vi "arduino_FSM.vi"() -> ()   [LabVIEW 2019]
uses:
  <vilib>/Instr/_visa.llb/VISA Configure Serial Port (Instr).vi
panel:
  out "Boolean":bool
  out "Waveform Chart":dbl(graph)
  out "Response":string
  in  "Output Current [A]":dbl(knob) max=1.0 scale=0.0..1.0 scale format="%#_4g"
  in  "Output Voltage [V]":dbl(knob) max=12.0 scale=12.0..15.0
  in  "DC Power Supply Settings":T1 {"Range" items=["P25V", "P6V", "N25V"]}
  in  "STOP":bool
  in  "Command":string="*IDN?"
  in  "Read Count":u32=1000
  in  "Write":bool
  in  "Read":bool
  in  "Serial Communication Settings":T2={"Port"="", "baud rate"=9600} {"baud rate" items=["75"=75, "110"=110, "134"=134, "150"=150, "300"=300, "600"=600, "1200"=1200, "1800"=1800, "2400"=2400, "4800"=4800, "7200"=7200, "9600"=9600, "14400"=14400, "19200"=19200, "28800"=28800, "38400"=38400, "56000"=56000, "57600"=57600, "115200"=115200, "128000"=128000, "230400"=230400]}
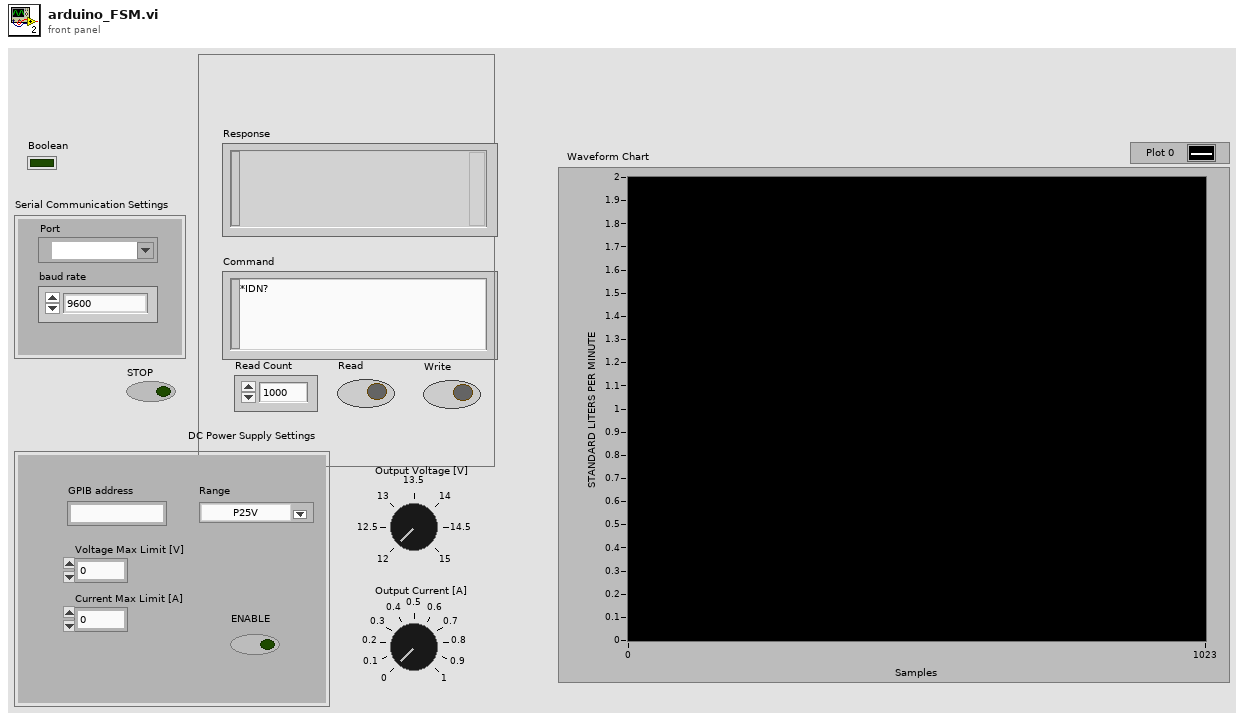
[diagram p1: front panel]
types:
  T1 = cluster{"GPIB address":string, "Range":u16, "Voltage Max Limit [V]":dbl, "Current Max Limit [A]":dbl, "ENABLE":bool}
  T2 = cluster{"Port":refnum<visa-resource-name>, "baud rate":u32}
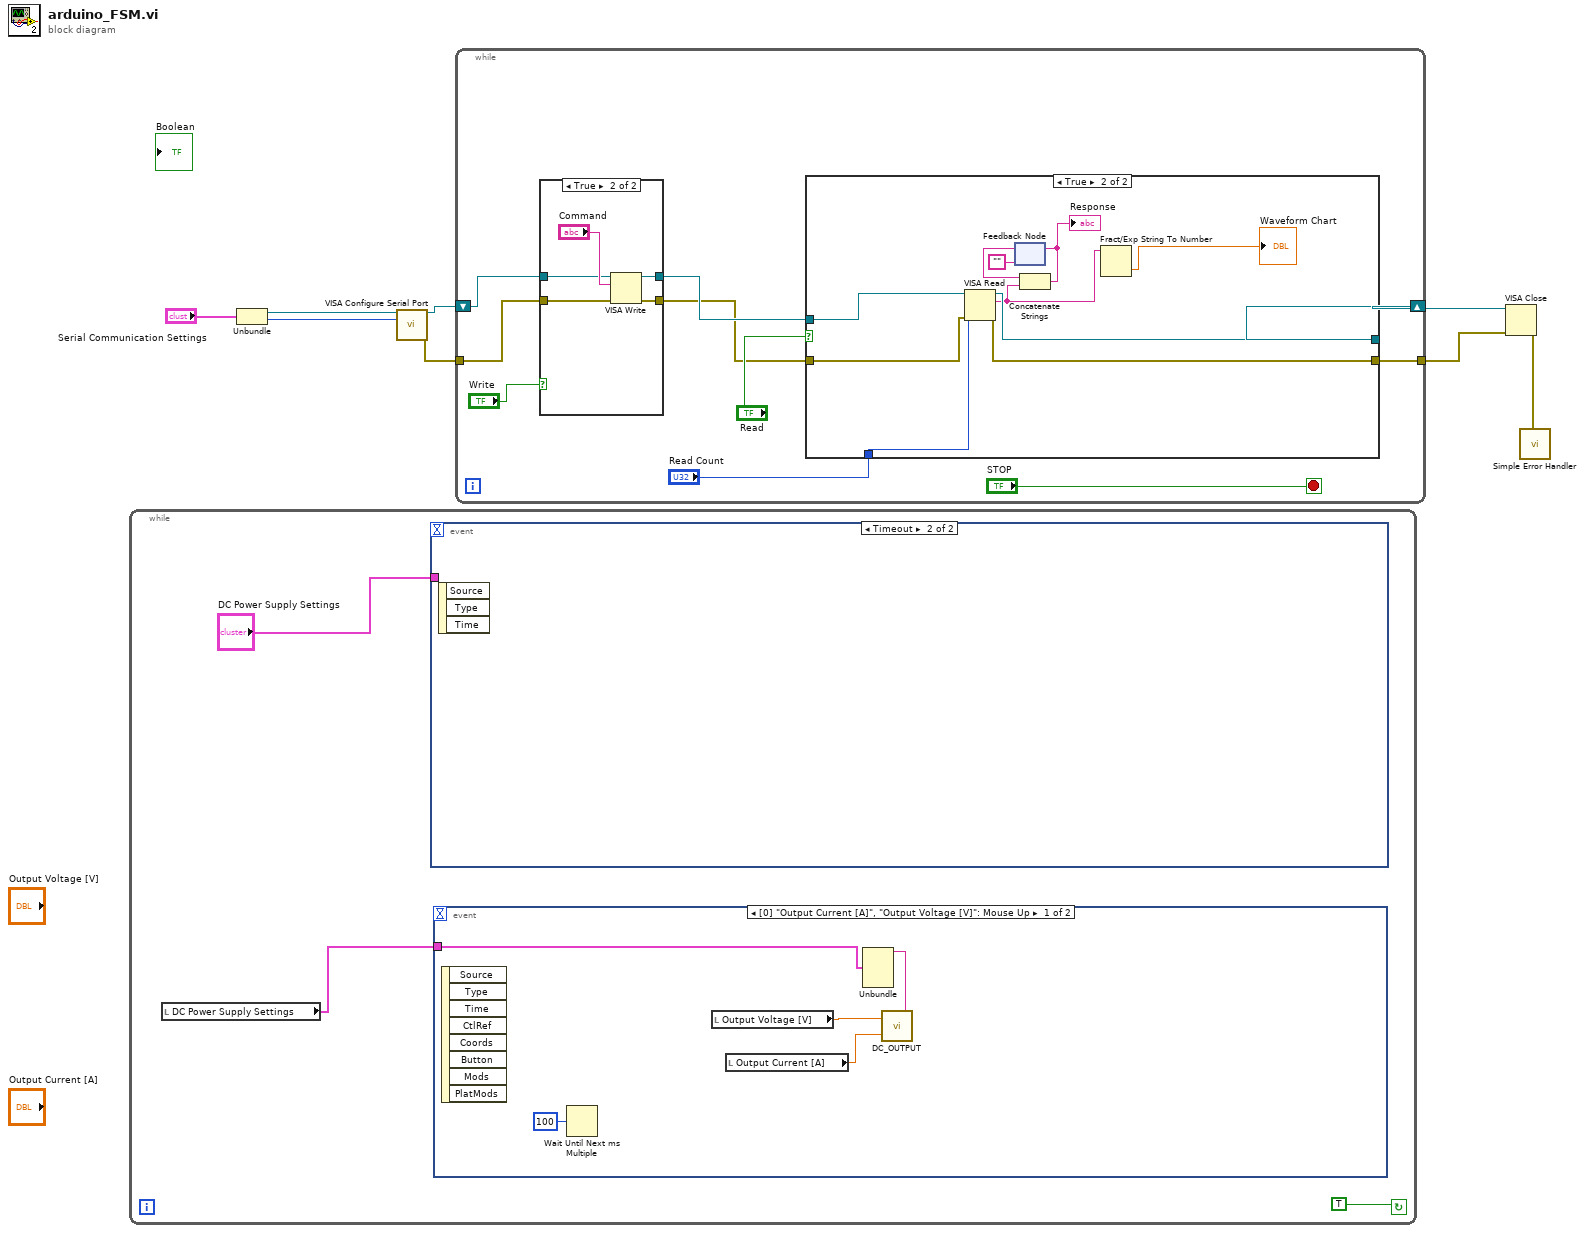
[diagram p0: block diagram]
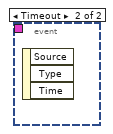
[diagram p2: hidden frame]
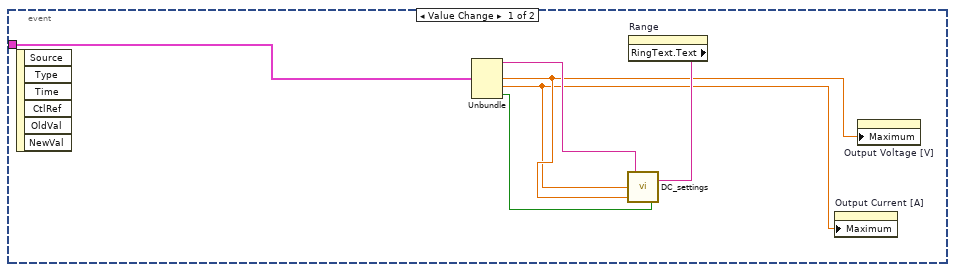
[diagram p3: hidden frame]
diagram:
  n1 = while {
    stop <- TRUE continue-if-true
    n2 = local read "DC Power Supply Settings"() -> (w10:T1)
    n3 = event shown="[1] Timeout" {
      selector: _ -> [_ _]
      dyn-events: _ -> [_ _]
      timeout: _ -> [_ _]
      tunnel: "DC Power Supply Settings" -> [w17 _]
      event "DC Power Supply Settings.ENABLE": Value Change {
        n4 = event-data() -> ()  [unwired: 1 in, 6 out]
        n5 = Unbundle(w17) -> ("GPIB address"=w22:string, "Voltage Max Limit [V]"=w20:dbl, "Current Max Limit [A]"=w19:dbl, "ENABLE"=w18:bool)  [unwired: 1 out]
        n6 = property on="Range" class="Ring (strict)"() -> ("RingText.Text"=w21:string)  [unwired: 2 in, 2 out]
        n7 = call "DC_settings.vi"("ENABLE"=w18, "Select Range"=w21, "Voltage Limit [V]"=w20, "Current Limit [A]"=w19, "E3631a address"=w22) -> ()
        n8 = property on="Output Current [A]" class="Knob (strict)"("Maximum"=w19) -> ()  [unwired: 2 in, 2 out]
        n9 = property on="Output Voltage [V]" class="Knob (strict)"("Maximum"=w20) -> ()  [unwired: 2 in, 2 out]
      }
      event Timeout {
        n10 = event-data() -> ()  [unwired: 1 in, 3 out]
      }
    }
    n11 = event shown="[0] \"Output Current [A]\", \"Output Voltage [V]\": Mouse Up" {
      selector: _ -> [_ _]
      dyn-events: _ -> [_ _]
      timeout: _ -> [_ _]
      tunnel: w10 -> [w15 _]
      event "Output Current [A]", "Output Voltage [V]": Mouse Up {
        n12 = event-data() -> ()  [unwired: 1 in, 8 out]
        n13 = Wait Until Next ms Multiple(millisecond multiple=u32 100) -> ()  [unwired: 1 out]
        n14 = local read "Output Voltage [V]"() -> (w14:dbl)
        n15 = local read "Output Current [A]"() -> (w13:dbl)
        n16 = Unbundle(w15) -> ("GPIB address"=w16:string)  [unwired: 4 out]
        n17 = call "DC_OUTPUT.vi"("String"=w16, "Current Output [A]"=w13, "Voltage Output [V]"=w14) -> ()
      }
      event Timeout {
        n18 = event-data() -> ()  [unwired: 1 in, 3 out]
      }
    }
  }
  n19 = Unbundle("Serial Communication Settings") -> ("Port"=w6:refnum<visa-resource-name>, "baud rate"=w7:u32)
  n20 = call-poly "VISA Configure Serial Port"("VISA resource name"=w6, "baud rate (9600)"=w7) -> ("VISA resource name out"=w4:refnum<visa-resource-name>, "error out"=w5:errorcluster)  [unwired: 8 in, 4 out]
  n21 = while {
    tunnel: w5 -> [w32]
    shift-right: [w26] -> w2
    shift-left: w4 -> [w25]
    tunnel: [w23] -> w3
    stop <- "STOP" stop-if-true
    n22 = case shown="True" "Write" {
      tunnel: w32 -> [w46 w51]
      tunnel: [w45 w50] -> w29
      tunnel: [w46 w49] -> w27
      tunnel: w25 -> [w45 w47]
      frame False {
      }
      frame True {
        n23 = VISA Write(VISA resource name=w47, write buffer="Command", error in (no error)=w51) -> (VISA resource name out=w50:refnum<visa-resource-name>, error out=w49:errorcluster)  [unwired: 1 out]
      }
    }
    n24 = case shown="True" "Read" {
      tunnel: w29 -> [w34 w41]
      tunnel: "Read Count" -> [_ w37]
      tunnel: w27 -> [w33 w40]
      tunnel: [w34 w38] -> w26
      tunnel: [w33 w39] -> w23
      frame False {
      }
      frame True {
        n25 = VISA Read(VISA resource name=w41, byte count=w37, error in (no error)=w40) -> (VISA resource name out=w38:refnum<visa-resource-name>, read buffer=w36:string, error out=w39:errorcluster)  [unwired: 1 out]
        n26 = feedback #1("") -> (w44:string)
        n27 = Concatenate Strings(w44, w36) -> (w43:string)
        "Response" <- w43
        n28 = feedback-in #1(w43) -> ()
        n29 = Fract/Exp String To Number(string=w36) -> (number=→"Waveform Chart":dbl)  [unwired: 3 in, 1 out]
      }
    }
  }
  n30 = VISA Close(VISA resource name=w2, error in (no error)=w3) -> (error out=w1:errorcluster)
  n31 = call <vilib>:"Simple Error Handler.vi"("error in (no error)"=w1) -> ()  [unwired: 1 in, 8 out]
